vi "WC_Drive_MotionMagic_DriveMotors.vi"(5 "Max Velocity":dbl, 7 "Cruise RPM":dbl, 8 "Error":errorcluster, 9 "RightSpeed":dbl, 10 "LeftSpeed":dbl, 11 "RobotDriveDevRef":T1={"DevStatus"={"status"=FALSE, "code"=0, "source"=""}, "Motors[]"=[], "Square Inputs"=FALSE, "Max Output"=1.0}) -> (0 "Error Out":errorcluster, 3 "RobotDriveDevRef Out":T1={"DevStatus"={"status"=FALSE, "code"=0, "source"=""}, "Motors[]"=[], "Square Inputs"=FALSE, "Max Output"=1.0})   [LabVIEW 2016]
doc: "Determines the motor configuration and sends the speed values to the appropriate motors.\n\nThis software is licensed. Open the labview\\readme\\WPI Robotics Library Open Source License.txt file for more information."
uses:
  <vilib>/Rock Robotics/WPI/RobotDrive/WPI_RobotDriveDevRef.ctl
  <vilib>/Rock Robotics/WPI/MotorControl/WPI_MotorControlDeviceRef.ctl
  <vilib>/Rock Robotics/WPI/MotorControl/WPI_MotorControlType.ctl
  <vilib>/Rock Robotics/SystemInterfaces/DIO/FPGA_DIOPWMChannel.ctl
  <vilib>/Rock Robotics/WPI/PWM/WPI_PWMDeadband.ctl
  <vilib>/Rock Robotics/WPI/ThirdParty/CanMotor/TalonSRX/WPI_CANTalonSRX_APIControlMode.ctl
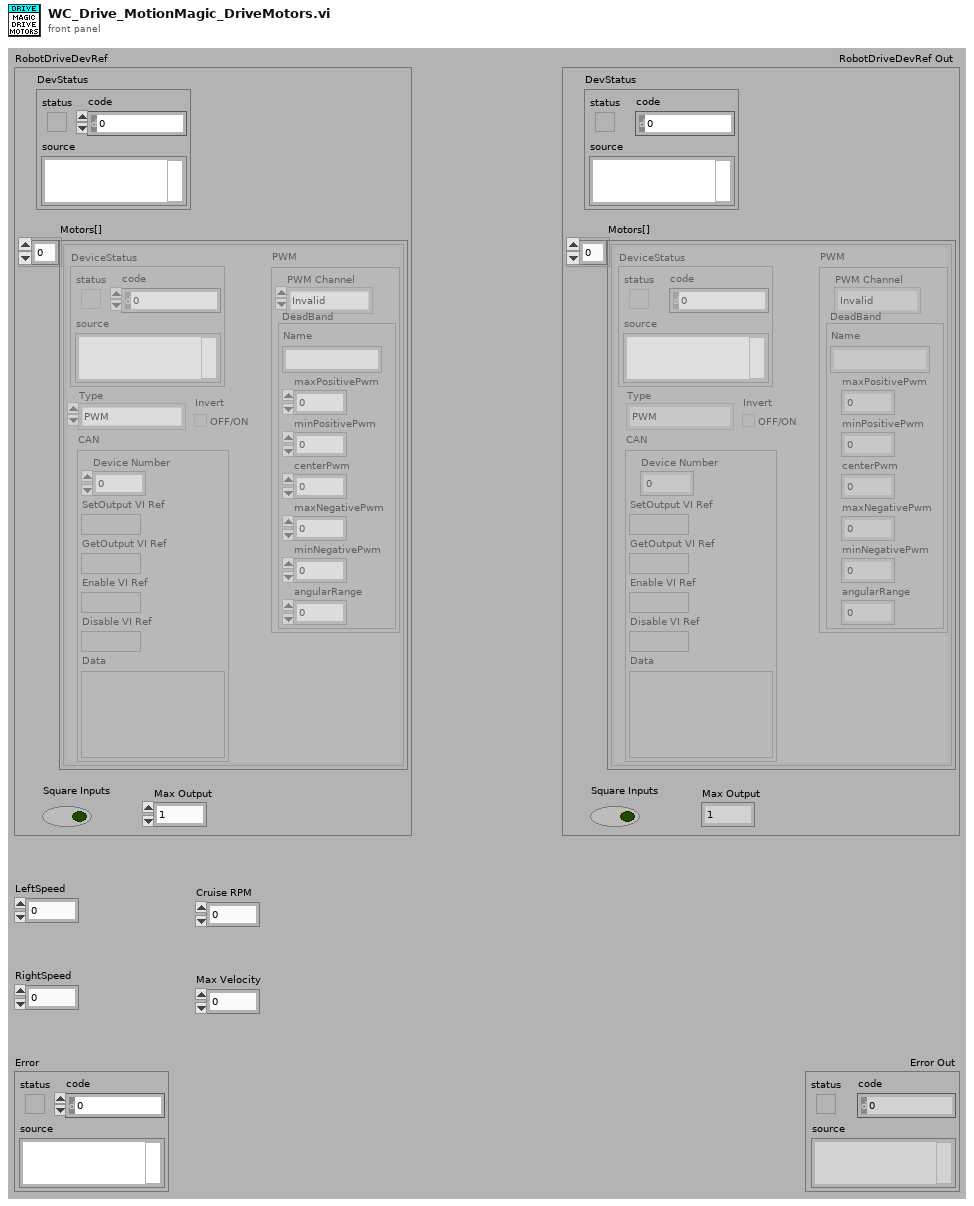
[diagram p1: front panel]
types:
  T1 = typedef "WPI_RobotDriveDevRef.ctl" = cluster{"DevStatus":errorcluster, "Motors[]":T2[], "Square Inputs":bool, "Max Output":dbl}
  T2 = typedef "WPI_MotorControlDeviceRef.ctl" = cluster{"DeviceStatus":errorcluster, "Type":T3, "PWM":cluster{"PWM Channel":T4, "DeadBand":T5}, "CAN":cluster{"Device Number":u8, "SetOutput VI Ref":variant, "GetOutput VI Ref":variant, "Enable VI Ref":variant, "Disable VI Ref":variant, "Data":variant}, "Invert":bool}
  T3 = typedef "WPI_MotorControlType.ctl" = enum16{"PWM", "CAN"}
  T4 = typedef "FPGA_DIOPWMChannel.ctl" = enum8{"PWM 0", "PWM 1", "PWM 2", "PWM 3", "PWM 4", "PWM 5", "PWM 6", "PWM 7", "PWM 8", "PWM 9", "PWM MXP 0", "PWM MXP 1", "PWM MXP 2", "PWM MXP 3", "PWM MXP 4", "PWM MXP 5", "PWM MXP 6", "PWM MXP 7", "PWM MXP 8", "PWM MXP 9", "Invalid"}
  T5 = typedef "WPI_PWMDeadband.ctl" = cluster{"Name":string, "maxPositivePwm":i32, "minPositivePwm":i32, "centerPwm":i32, "maxNegativePwm":i32, "minNegativePwm":i32, "angularRange":u16}
  T6 = typedef "WPI_CANTalonSRX_APIControlMode.ctl" = enum8{"Percent VBus", "Speed", "Position", "Slave", "Unchanged / Invalid", "Voltage Compensation", "Current", "Motion Profile", "Motion Magic"}
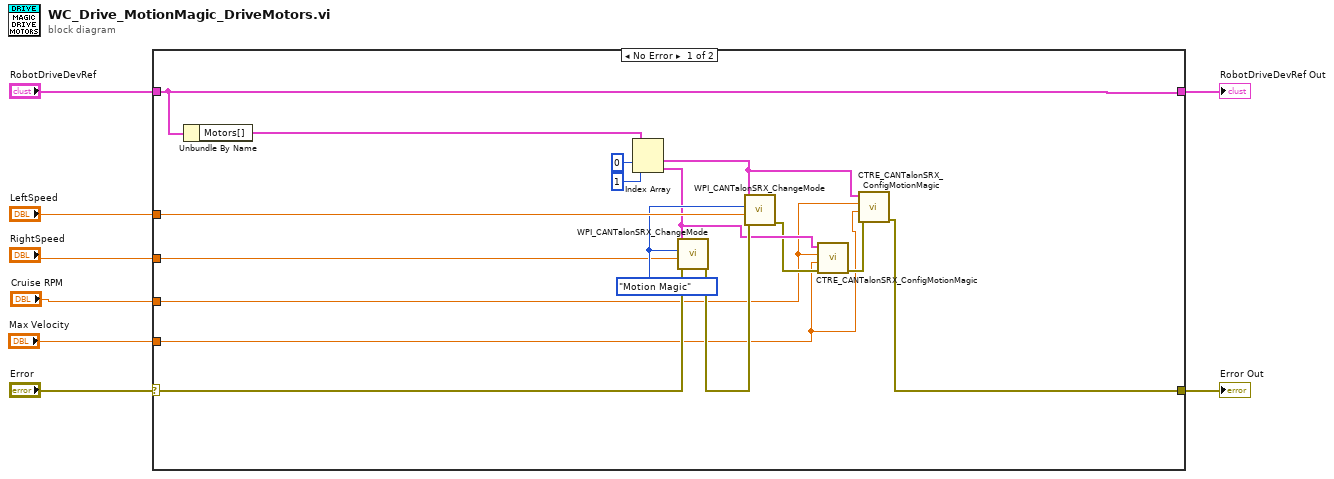
[diagram p0: block diagram]
diagram:
  n1 = case shown="No Error" "Error" {
    selector: "Error" -> [w17 w26]
    tunnel: "RobotDriveDevRef" -> [w18 w25]
    tunnel: [w18 w25] -> w7
    tunnel: "LeftSpeed" -> [w21 _]
    tunnel: "RightSpeed" -> [w19 _]
    tunnel: [w11 w26] -> w3
    tunnel: "Cruise RPM" -> [w10 _]
    tunnel: "Max Velocity" -> [w9 _]
    frame No Error {
      w20 = WPI_CANTalonSRX_APIControlMode."Motion Magic" ("Control Mode")
      n2 = Unbundle By Name(w18) -> ("Motors[]"=w22:T2[])
      n3 = Index Array(array=w22, index #1=0 ("index"), index #2=1 ("index")) -> (element #1=w14:T2, element #2=w15:T2)
      n4 = call <vilib>:"WPI_CANTalonSRX_ChangeMode.vi"("error in (no error)"=w17, "Output"=w19, "Control Mode"=w20, "CAN Talon SRX Ref"=w15) -> ("error out"=w16:errorcluster)  [unwired: 6 in, 1 out]
      n5 = call <vilib>:"WPI_CANTalonSRX_ChangeMode.vi"("error in (no error)"=w16, "Output"=w21, "Control Mode"=w20, "CAN Talon SRX Ref"=w14) -> ("error out"=w13:errorcluster)  [unwired: 6 in, 1 out]
      n6 = call <vilib>:"CTRE_CANTalonSRX_ConfigMotionMagic.vi"("error in (no error)"=w13, "Max Acceleration"=w9, "Cruise Velocity"=w10, "CAN Talon SRX Ref"=w15) -> ("error out"=w12:errorcluster)  [unwired: 6 in, 1 out]
      n7 = call <vilib>:"CTRE_CANTalonSRX_ConfigMotionMagic.vi"("error in (no error)"=w12, "Max Acceleration"=w9, "Cruise Velocity"=w10, "CAN Talon SRX Ref"=w14) -> ("error out"=w11:errorcluster)  [unwired: 6 in, 1 out]
    }
    frame Error {
    }
  }
  "RobotDriveDevRef Out" <- w7
  "Error Out" <- w3
